vi "New.vi"   [LabVIEW 2021]
uses:
  RSA/RSA.lvclass
  AES/AES.lvclass
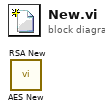
[diagram p0: block diagram]
diagram:
  n1 = call "AES New.vi"() -> ()  [unwired: 10 in, 2 out]
  n2 = call "RSA New.vi"() -> ()  [unwired: 10 in, 2 out]
